vi "AlliGator Load Calibration Phasor.vi"(8 "Error In":errorcluster, 10 "File Path":path, 11 "Calibration Phasor in":T1) -> (0 "error out":errorcluster, 1 "Phasor Frequency":dbl[unit], 2 "XML File Path":path, 3 "Calibration Phasor out":T1, 4 "Message":string)   [LabVIEW 2021, in "AlliGator Phasor Calibration.lvlib"]
doc: "Loads a <B>Calibration Phasor</B>."
uses:
  AlliGator Phasor Calibration.lvlib
  Phasor/Calibration Phasor (m, phi).ctl
  dc872a39-2f0f-422b-bdbb-2959c88d23f9.vi
  dc872a39-2f0f-422b-bdbb-2959c88d23f9.vi/8a80743f-1319-44c8-96b0-3ef8fc688731.vi
  dc872a39-2f0f-422b-bdbb-2959c88d23f9.vi/931f4f8f-d8c6-4056-833f-5c8fe97b24b9.vi
  <vilib>/Utility/error.llb/Error Cluster From Error Code.vi
  <vilib>/ErrorRing/Error Ring.xnode
  Files/Files.lvlib
  Phasor/Phasor.lvlib
  Settings/AlliGator Settings.lvlib
panel:
  # "see the AlliGator License on the block diagram (Ctrl+E or Window:Show Block Diagram)"
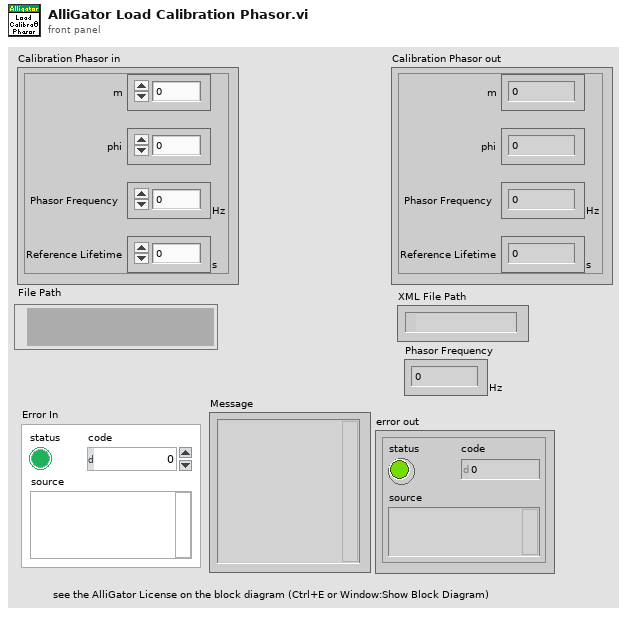
[diagram p1: front panel]
types:
  T1 = typedef "Phasor.lvlib/Calibration Phasor (m, phi).ctl" = cluster{"m":dbl, "phi":dbl, "Phasor Frequency":dbl[unit], "Reference Lifetime":dbl[unit]}
  T2 = typedef "Phasor.lvlib/Phasor (g, s).ctl" = cluster{"g":dbl, "s":dbl}
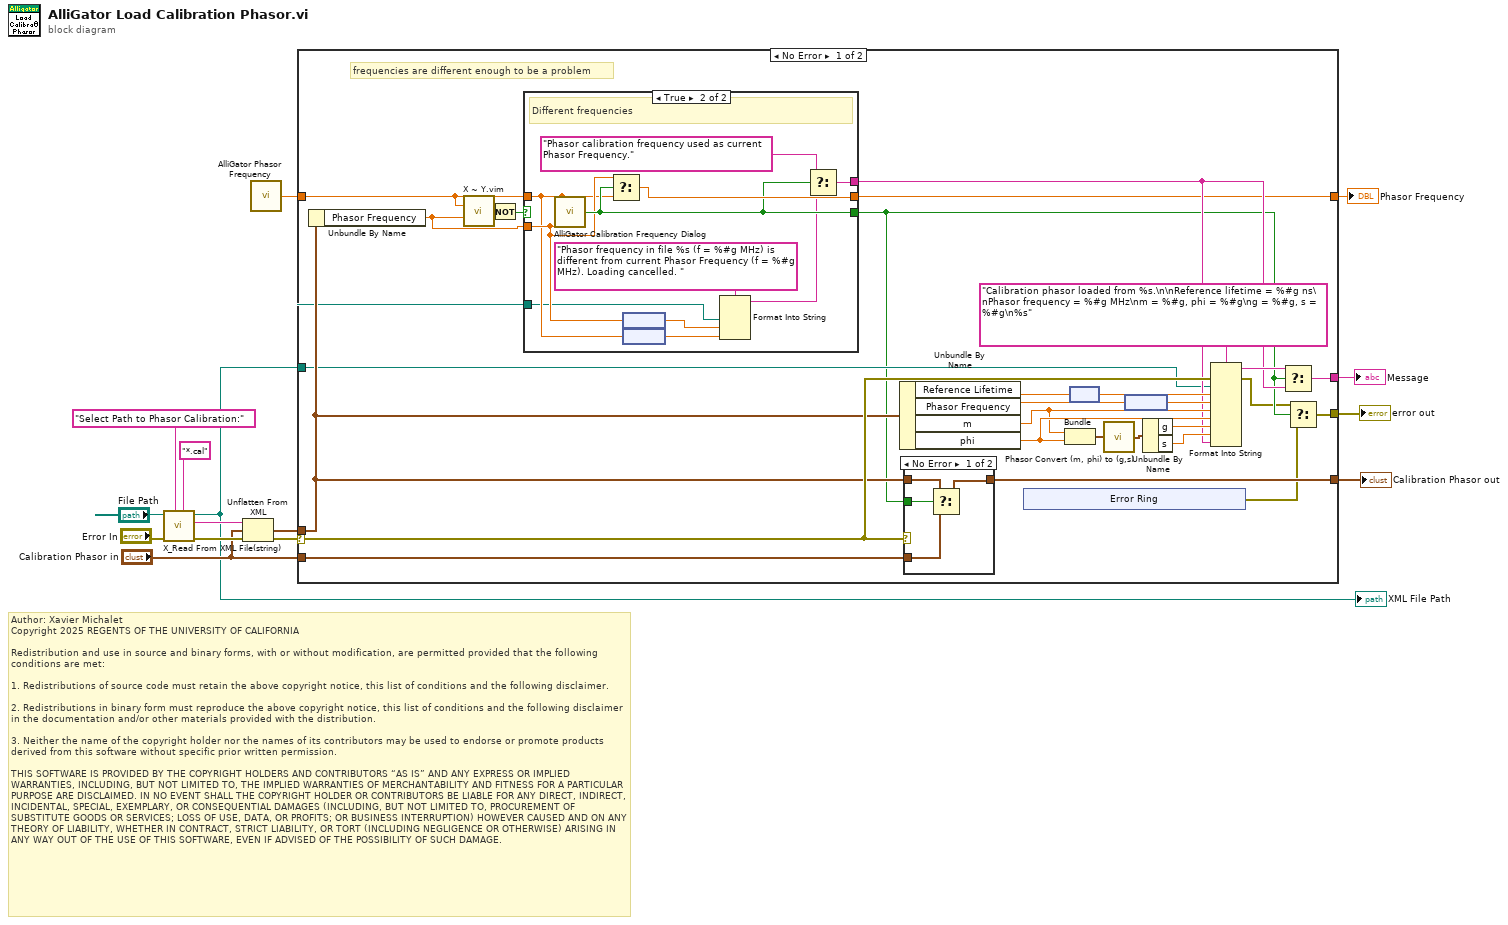
[diagram p0: block diagram]
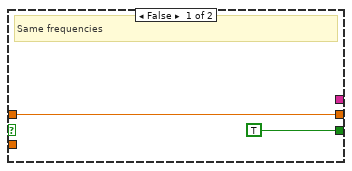
[diagram p3: hidden frame]
diagram:
  # "Author: Xavier Michalet\nCopyright 2025 REGENTS OF THE UNIVERSITY OF CALIFORNIA\n\nRedistribution and use in source and binary forms, with or without modification, are permitted provided that the following conditions are met:\n\n1. Redistributions of source code must retain the above copyright notice, this list of conditions and the following disclaimer.\n\n2. Redistributions in binary form must reproduce the above copyright notice, this list of conditions and the following disclaimer in the documentation and/or other materials provided with the distribution.\n\n3. Neither the name of the copyright holder nor the names of its contributors may be used to endorse or promote products derived from this software without specific prior written permission.\n\nTHIS SOFTWARE IS PROVIDED BY THE COPYRIGHT HOLDERS AND CONTRIBUTORS “AS IS” AND ANY EXPRESS OR IMPLIED WARRANTIES, INCLUDING, BUT NOT LIMITED TO, THE IMPLIED WARRANTIES OF MERCHANTABILITY AND FITNESS FOR A PARTICULAR PURPOSE ARE DISCLAIMED. IN NO EVENT SHALL THE COPYRIGHT HOLDER OR CONTRIBUTORS BE LIABLE FOR ANY DIRECT, INDIRECT, INCIDENTAL, SPECIAL, EXEMPLARY, OR CONSEQUENTIAL DAMAGES (INCLUDING, BUT NOT LIMITED TO, PROCUREMENT OF SUBSTITUTE GOODS OR SERVICES; LOSS OF USE, DATA, OR PROFITS; OR BUSINESS INTERRUPTION) HOWEVER CAUSED AND ON ANY THEORY OF LIABILITY, WHETHER IN CONTRACT, STRICT LIABILITY, OR TORT (INCLUDING NEGLIGENCE OR OTHERWISE) ARISING IN ANY WAY OUT OF THE USE OF THIS SOFTWARE, EVEN IF ADVISED OF THE POSSIBILITY OF SUCH DAMAGE."
  n1 = call "X_Read From XML File(string).vi"("pattern (*.xml)"="*.cal", "Prompt"="Select Path to Phasor Calibration:", "error in (no error)"="Error In", "XML File Path"="File Path") -> ("error out"=w15:errorcluster, "XML Elements"=w14:string, "XML File Path(duplicate)"=w4:path)  [unwired: 5 in]
  "XML File Path" <- w4
  n2 = Unflatten From XML(xml string=w14, type="Calibration Phasor in", error in (no error)=w15) -> (value=w7:T1, error out=w8:errorcluster)
  n3 = call "AlliGator Phasor Frequency.vi"() -> ("Phasor Frequency"=w1:dbl[unit])
  n4 = case shown="No Error" w8 {
    selector: w8 -> [w30 w68]
    tunnel: [w42 w67] -> w11
    tunnel: w7 -> [w27 _]
    tunnel: "Calibration Phasor in" -> [w26 w67]
    tunnel: [w24 _] -> w5
    tunnel: w4 -> [w22 _]
    tunnel: [w21 w66] -> w3
    tunnel: [w18 w68] -> w2
    tunnel: w1 -> [w16 w66]
    frame No Error {
      # "frequencies are different enough to be a problem"
      n5 = Unbundle By Name(w27) -> ("Phasor Frequency"=w28:dbl[unit])
      n6 = call "X ~ Y.vim"("X"=w16, "Y"=w28) -> ("X ~= Y?"=w43:bool)  [unwired: 13 in]
      n7 = Not(x=w43) -> (.not. x?=w29:bool)
      n8 = case shown="True" w29 {
        tunnel: w16 -> [w54 w57]
        tunnel: w28 -> [_ w59]
        tunnel: [TRUE ("Use Calibration Frequency?") w63] -> w20
        tunnel: [w54 w65] -> w21
        tunnel: [_ w62] -> w23
        tunnel: w22 -> [_ w55]
        frame False {
          # "Same frequencies"
        }
        frame True {
          # "Different frequencies"
          n9 = call "AlliGator Calibration Frequency Dialog.vi"("Calibration Phasor Frequency"=w59, "Internal Phasor Frequency"=w57) -> ("Use Calibration Frequency?"=w63:bool)
          n10 = Select(t=w59, s=w63, f=w57) -> (s? t:f=w65:dbl[unit])
          n11 = node(w59) -> (w61:dbl)
          n12 = node(w57) -> (w58:dbl)
          n13 = Format Into String(format string="Phasor frequency in file %s (f = %#g MHz) is different from current Phasor Frequency (f = %#g MHz). Loading cancelled. ", w55, w61, w58) -> (resulting string=w56:string)  [unwired: 2 in, 1 out]
          n14 = Select(t="Phasor calibration frequency used as current Phasor Frequency." ("format string"), s=w63, f=w56) -> (s? t:f=w62:string)
        }
      }
      n15 = Unbundle By Name(w27) -> ("Reference Lifetime"=w35:dbl[unit], "Phasor Frequency"=w34:dbl[unit], "m"=w36:dbl, "phi"=w41:dbl)
      n16 = case shown="No Error" w30 {
        tunnel: w27 -> [w50 w52]
        tunnel: [w48 w52] -> w42
        tunnel: w26 -> [w49 _]
        tunnel: w20 -> [w51 _]
        frame No Error {
          n17 = Select(t=w50, s=w51, f=w49) -> (s? t:f=w48:T1)
        }
        frame Error {
        }
      }
      n18 = xnode "Error Ring"() -> ("error out"=w17:errorcluster)
      n19 = Bundle("m"=w36, "phi"=w41) -> (w40:cluster{"m":dbl, "phi":dbl})  [unwired: 1 in]
      n20 = node(w35) -> (w33:dbl)
      n21 = call "Phasor Convert (m, phi) to (g,s).vi"("Phasor (m, phi)"=w40) -> ("Phasor (g, s)"=w39:T2)  [unwired: 8 in]
      n22 = node(w34) -> (w32:dbl)
      n23 = Unbundle By Name(w39) -> ("g"=w38:dbl, "s"=w37:dbl)
      n24 = Format Into String(format string="Calibration phasor loaded from %s.\n\nReference lifetime = %#g ns\nPhasor frequency = %#g MHz\nm = %#g, phi = %#g\ng = %#g, s = %#g\n%s", error in=w30, w22, w33, w32, w36, w41, w38, w37, w23) -> (resulting string=w25:string, error out=w19:errorcluster)  [unwired: 1 in]
      n25 = Select(t=w25, s=w20, f=w23) -> (s? t:f=w24:string)
      n26 = Select(t=w19, s=w20, f=w17) -> (s? t:f=w18:errorcluster)
    }
    frame Error {
    }
  }
  "Calibration Phasor out" <- w11
  "error out" <- w2
  "Message" <- w5
  "Phasor Frequency" <- w3
